vi "Update Bus A Pointers.vi"(8 "error in (no error)":errorcluster, 9 "Data Pointers":u16[](array[numeric]) format="%.0x", 10 "Command Words":u16[](array[numeric]) format="%.0x", 11 "Bus Monitor in":refnum<class "Bus Monitor.lvclass">) -> (0 "error out":errorcluster, 3 "Bus Monitor out":refnum<class "Bus Monitor.lvclass">)   [LabVIEW 2020, in "BCI-1553 API.lvlib" / "Bus Monitor.lvclass"]
doc: "Reads all the Bus A filters and updates their data pointers. If there is still a valid or new data pointer in memory for the filter parameters, they receive that pointer. If there is no command in memory, the parameter data pointer is set to zero. Zero is used as a flag for later to indicate a no change in data."
uses:
  Bus Monitor.lvclass
  Bus Monitor.lvclass/Bus Monitor.ctl
  Dependencies/Registry/Registry.lvclass/Registry.ctl
  Filters/Filter/Filter.lvclass
  Dependencies/Registry/Registry.lvclass
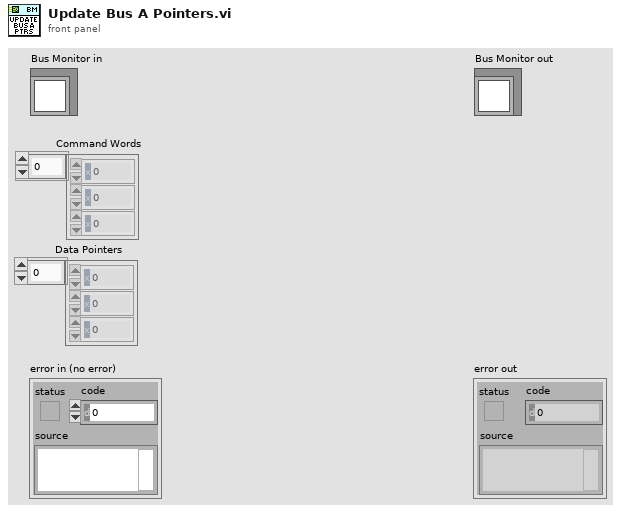
[diagram p1: front panel]
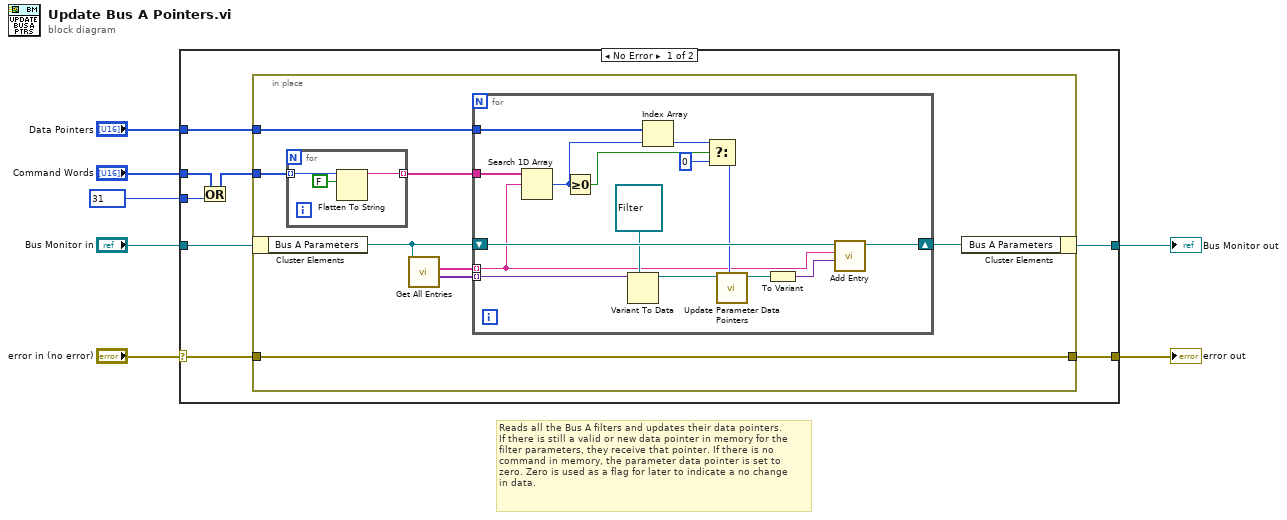
[diagram p0: block diagram]
diagram:
  # "Reads all the Bus A filters and updates their data pointers.\nIf there is still a valid or new data pointer in memory for the\nfilter parameters, they receive that pointer. If there is no\ncommand in memory, the parameter data pointer is set to\nzero. Zero is used as a flag for later to indicate a no change\nin data."
  n1 = case shown="No Error" "error in (no error)" {
    selector: "error in (no error)" -> [w11 w43]
    tunnel: [w12 w43] -> w6
    tunnel: [w13 w42] -> w4
    tunnel: "Bus Monitor in" -> [w14 w42]
    tunnel: "Command Words" -> [w9 _]
    tunnel: "Data Pointers" -> [w15 _]
    tunnel: u16 31 -> [w10 _]
    frame No Error {
      n2 = Or(x=w9, y=w10) -> (x .or. y?=w8:u16[])
      n3 = in-place {
        in-place-border: w8 -> [w22]
        in-place-border: w15 -> [w16]
        in-place-border: [w23] -> w12
        in-place-border: w11 -> [w23]
        n4 = in-place-cluster #1(w14) -> ("Bus A Parameters"=w19:refnum<class "Registry.lvclass">)
        n5 = for {
          tunnel: w22 -> [w41] mode=indexing
          tunnel: [w39] -> w17 mode=indexing
          n6 = Flatten To String(anything=w41, prepend array or string size? (T)=FALSE) -> (data string=w39:string)  [unwired: 2 in, 2 out]
        }
        n7 = call "Get All Entries.vi"("Registry in"=w19) -> ("Values"=w20:variant[], "Keys"=w21:string[])  [unwired: 8 in, 1 out]
        n8 = for {
          tunnel: w21 -> [w24] mode=indexing
          tunnel: w20 -> [w33] mode=indexing
          shift-right: [w38] -> w18
          shift-left: w19 -> [w37]
          tunnel: w17 -> [w36]
          tunnel: w16 -> [w35]
          n9 = Search 1D Array(1D array=w36, element=w24) -> (index of element=w34:i32)  [unwired: 1 in]
          n10 = Greater Or Equal To 0?(x=w34) -> (x >= 0?=w30:bool)
          n11 = Variant To Data(type=refnum<class "Filter.lvclass"> refnum ("SLSC 1553 API.lvlib:Filter.lvclass"), Variant=w33) -> (data=w31:refnum<class "Filter.lvclass">)  [unwired: 1 in, 1 out]
          n12 = Index Array(array=w35, index=w34) -> (element=w29:u16)
          n13 = Select(t=w29, s=w30, f=u16 0) -> (s? t:f=w27:u16)
          n14 = call-dynamic "Update Parameter Data Pointers.vi"("Data Pointer"=w27, "Filter in"=w31) -> ("Filter out"=w26:refnum<class "Filter.lvclass">)  [unwired: 8 in, 1 out]
          n15 = To Variant(anything=w26) -> (Variant=w25:variant)
          n16 = call "Add Entry.vi"("Value"=w25, "Key"=w24, "Registry in"=w37) -> ("Registry out"=w38:refnum<class "Registry.lvclass">)  [unwired: 6 in, 2 out]
        }
        n17 = in-place-cluster #1("Bus A Parameters"=w18) -> (w13:refnum<class "Bus Monitor.lvclass">)
      }
    }
    frame Error {
    }
  }
  "error out" <- w6
  "Bus Monitor out" <- w4
